vi "PCIe SLM - Calculate Image.vi"(8 "error in (no error)":errorcluster, 9 "Supress Ghost Orders":bool, 11 "Spots, Params and Zernike":T5 {"Spots"."Spot Params"."Z" format="%_4g"; "Spots"."Spot Params"."Y" format="%_4g"; "Spots"."Spot Params"."X" format="%_4g"; "Spots"."Spot Params"."Phase" format="%_4g"; "Spots"."Spot Params"."Intensity" format="%_4g"; "SLM Parameters"."Centre X" format="%.3g"; "SLM Parameters"."Centre Y" format="%.3g"; "Zernikes"."SecComaY" step=0.01; "Zernikes"."SecComaX" step=0.01; "Zernikes"."SecAstigY" step=0.01; "Zernikes"."SecAstigX" step=0.01; "Zernikes"."ComaY" step=0.01; "Zernikes"."ComaX" step=0.01; "Zernikes"."AstigY" step=0.01; "Zernikes"."AstigX" step=0.01}) -> (0 "error out":errorcluster)   [LabVIEW 2020]
doc: "Use this template to build a VI to use as a subVI."
uses:
  _controls/PCIe SLM Spots.ctl
  _controls/Spot Params.ctl
  _controls/PCIe SLM params.ctl
  _controls/PCIe SLM Zernike Coefs.ctl
  <userlib>/SLM Lib/SLM Lib.lvlib
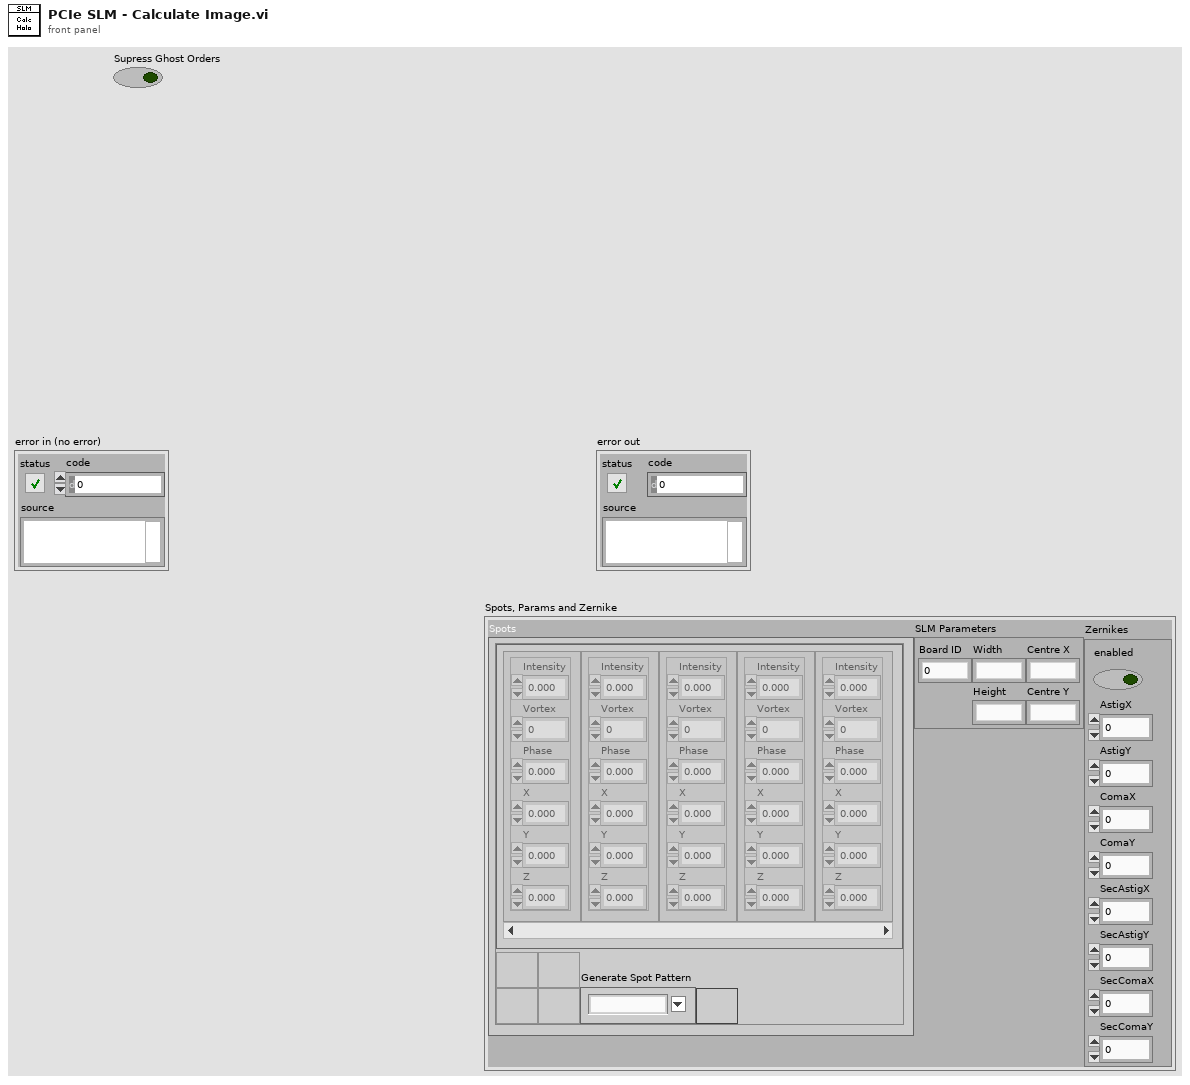
[diagram p1: front panel]
types:
  T1 = typedef "PCIe SLM Spots.ctl" = cluster{"Spot Params":T2, "Add Spot":bool, "Remove Spot":bool, "Clear All Spots":bool, "Save Spots":bool, "Generate Spots":bool, "Generate Spot Pattern":string}
  T2 = typedef "Spot Params.ctl" = cluster{"Intensity":dbl, "Vortex":dbl, "Phase":dbl, "X":dbl, "Y":dbl, "Z":dbl}[]
  T3 = typedef "PCIe SLM params.ctl" = cluster{"Width":dbl, "Height":dbl, "Board ID":i32, "Centre Y":dbl, "Centre X":dbl}
  T4 = typedef "PCIe SLM Zernike Coefs.ctl" = cluster{"enabled":bool, "AstigX":dbl, "AstigY":dbl, "ComaX":dbl, "ComaY":dbl, "SecAstigX":dbl, "SecAstigY":dbl, "SecComaX":dbl, "SecComaY":dbl}
  T5 = cluster{"Spots":T1, "SLM Parameters":T3, "Zernikes":T4}
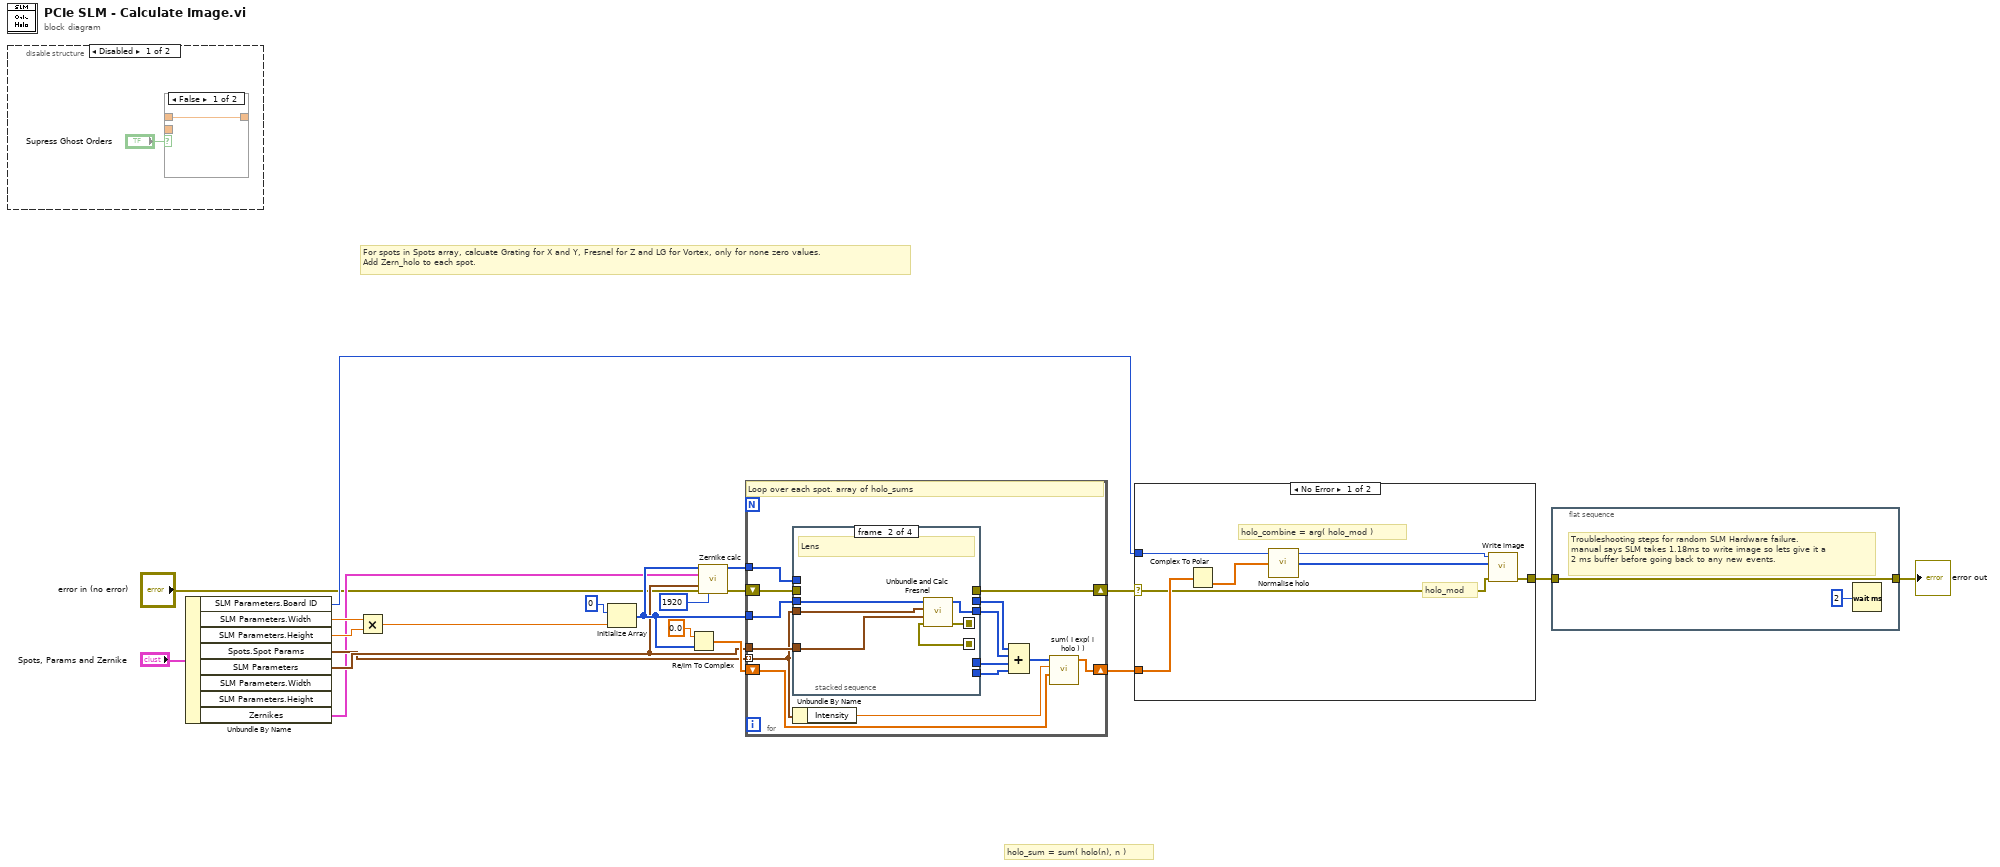
[diagram p0: block diagram]
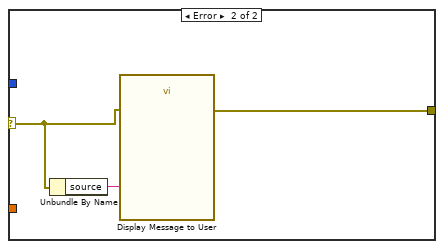
[diagram p2: hidden frame]
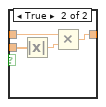
[diagram p3: hidden frame]
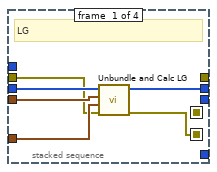
[diagram p5: hidden frame]
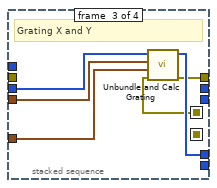
[diagram p6: hidden frame]
diagram:
  # "holo_sum = sum( holo(n), n )"
  # "For spots in Spots array, calcuate Grating for X and Y, Fresnel for Z and LG for Vortex, only for none zero values.\nAdd Zern_holo to each spot."
  n1 = disable-structure shown="Disabled" {
    frame Disabled {
      n2 = case shown="False" "Supress Ghost Orders" {
        tunnel: _ -> [w22 w25]
        tunnel: [w22 w24] -> _
        tunnel: _ -> [_ w23]
        frame False {
        }
        frame True {
          n3 = Absolute Value(x=w23) -> (abs(x)=w26:dbl)
          n4 = Multiply(x=w25, y=w26) -> (x*y=w24:dbl)
        }
      }
    }
    frame Enabled {
    }
  }
  n5 = Unbundle By Name("Spots, Params and Zernike") -> ("SLM Parameters.Board ID"=w8:i32, "SLM Parameters.Width"=w11:dbl, "SLM Parameters.Height"=w10:dbl, "Spots.Spot Params"=w9:T2, "SLM Parameters"=w12:T3, "Zernikes"=w6:T4)  [unwired: 2 out]
  n6 = Multiply(x=w11, y=w10) -> (x*y=w19:dbl)
  n7 = Initialize Array(u8 0 ("element"), w19) -> (w15:u8[])
  n8 = Re/Im To Complex(1:w15, 2:0.0 ("x")) -> (0:w17:cdb[])
  n9 = call "Zernike calc.vi"("holo_init"=w15, "Zernike Coefs Cluster"=w6, "SLM Params"=w12, "error in (no error)"="error in (no error)", "radius"=1920) -> ("Zernike holo"=w14:u8[], "error out"=w5:errorcluster)  [unwired: 9 in]
  n10 = for {
    tunnel: w9 -> [w29] mode=indexing
    tunnel: w15 -> [w40]
    shift-right: [w36] -> w16
    shift-left: w17 -> [w30]
    tunnel: w14 -> [w34]
    tunnel: w12 -> [w32]
    shift-right: [w27] -> w4
    shift-left: w5 -> [w28]
    # "Loop over each spot. array of holo_sums"
    n11 = stacked-sequence {
      seq-local: [w41 _ _ _] -> [_ w48 _ _]
      seq-local: [_ w47 _ _] -> [_ _ w54 _]
      tunnel: w40 -> [w46 w51 w57 _]
      tunnel: [w43 _ _ _] -> w39
      tunnel: [_ w52 _ _] -> w38
      tunnel: [_ _ w58 _] -> w37
      tunnel: [_ _ _ w59] -> w33
      tunnel: w34 -> [_ _ _ w59]
      tunnel: w32 -> [w45 w49 w55 _]
      tunnel: w29 -> [w44 w50 w56 _]
      tunnel: w28 -> [w42 _ _ _]
      tunnel: [_ _ w53 _] -> w27
      frame #0 {
        # "LG"
        n12 = call "Unbundle and Calc LG.vi"("error in (no error)"=w42, "SLM Params"=w45, "Spot Settings"=w44, "holo_init"=w46) -> ("error out"=w41:errorcluster, "LG holo"=w43:u8[])  [unwired: 6 in]
      }
      frame #1 {
        # "Lens"
        n13 = call "Unbundle and Calc Fresnel.vi"("error in (no error)"=w48, "SLM Params"=w49, "Spot Settings"=w50, "holo_init"=w51) -> ("error out"=w47:errorcluster, "Fresnel holo"=w52:u8[])  [unwired: 6 in]
      }
      frame #2 {
        # "Grating X and Y"
        n14 = call "Unbundle and Calc Grating.vi"("error in (no error)"=w54, "SLM Params"=w55, "Spot Settings"=w56, "holo_init"=w57) -> ("error out"=w53:errorcluster, "Grating Holo"=w58:u8[])  [unwired: 6 in]
      }
      frame #3 {
        # "Aberations"
      }
    }
    n15 = Unbundle By Name(w29) -> ("Intensity"=w31:dbl)
    n16 = Compound Arithmetic op=ADD(w39, w38, w37, w33) -> (w35:u8[])
    n17 = call "sum( I exp( i holo ) ).vi"("Spot(n-1) holo"=w30, "Spot(n) Intensity"=w31, "Spot(n) Holo"=w35) -> ("holo_mod"=w36:cdb[])  [unwired: 8 in]
  }
  n18 = case shown="No Error" w4 {
    selector: w4 -> [w61 w66]
    tunnel: w16 -> [w63 _]
    tunnel: w8 -> [w62 _]
    tunnel: [w60 w67] -> w1
    frame No Error {
      # "holo_mod"
      # "holo_combine = arg( holo_mod )"
      n19 = Complex To Polar(r * e^(i*theta)=w63) -> (theta=w64:dbl[])  [unwired: 1 out]
      n20 = call "Normalise holo.vi"("holo _comb in"=w64) -> ("holo_comb out"=w65:u8[])
      n21 = call <userlib>:"Write image.vi"("error in (no error)"=w61, "image"=w65, "board"=w62) -> ("error out"=w60:errorcluster)  [unwired: 6 in, 2 out]
    }
    frame Error {
      n22 = Unbundle By Name(w66) -> ("source"=w68:string)
      n23 = call "Display Message to User"("error in (no error)"=w66, "Message"=w68) -> ("error out"=w67:errorcluster)  [unwired: 8 in, 1 out]
    }
  }
  n24 = flat-sequence {
    tunnel: [w70] -> w2
    tunnel: w1 -> [w70]
    frame #0 {
      # "Troubleshooting steps for random SLM Hardware failure.\nmanual says SLM takes 1.18ms to write image so lets give it a \n2 ms buffer before going back to any new events."
      n25 = Wait (ms)(milliseconds to wait=u32 2) -> ()  [unwired: 1 out]
    }
  }
  "error out" <- w2
